vi "vipbBuild.vi"() -> ()   [LabVIEW 2014, in "lv-cli-steps.lvlib"]
uses:
  lv-cli-steps.lvlib
  <vilib>/Utility/error.llb/DialogType.ctl
  <vilib>/Wiresmith Technology/LabVIEW CLI/CLI Class/CLI.lvclass
  <vilib>/JKI/VIPM API/VIPM API_vipm_api.lvlib
panel:
  out "error out":errorcluster
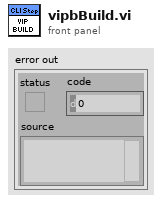
[diagram p1: front panel]
types:
  T1 = typedef "DialogType.ctl" = u16
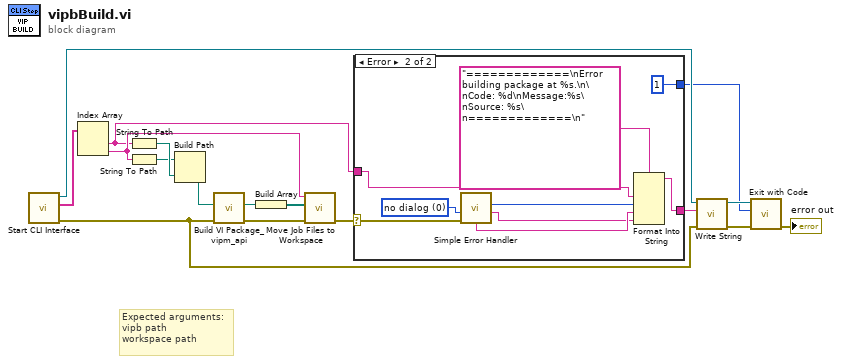
[diagram p0: block diagram]
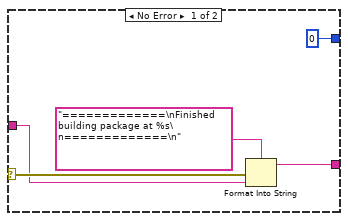
[diagram p2: hidden frame]
diagram:
  # "Expected arguments:\nvipb path\nworkspace path"
  n1 = call <vilib>:"Start CLI Interface.vi"() -> ("error out"=w3:errorcluster, "Custom Parameters"=w17:string[], "CLI out"=w15:refnum<class "CLI.lvclass">)  [unwired: 9 in]
  n2 = Index Array(array=w17) -> (element #1=w1:string, element #2=w7:string)  [unwired: 2 in]
  n3 = String To Path(string=w1) -> (path=w11:path)
  n4 = String To Path(string=w7) -> (path=w10:path)
  n5 = Build Path(base path=w10, name or relative path=w11) -> (appended path=w2:path)
  n6 = call <vilib>:"Build VI Package_vipm_api.vi"("error in (no error)"=w3, "Path to VIPB File"=w2) -> ("error out"=w4:errorcluster, "Build Output"=w6:path)  [unwired: 8 in]
  n7 = Build Array(w6) -> (w5:path[])
  n8 = call "Move Job Files to Workspace.vi"("error in (no error)"=w4, "Generated Files"=w5, "Workspace Path"=w7) -> ("error out"=w9:errorcluster)  [unwired: 8 in]
  n9 = case shown="Error" w9 {
    selector: w9 -> [w21 w30]
    tunnel: w1 -> [w20 w26]
    tunnel: [w19 w31] -> w16
    tunnel: [0 ("Exit Code (0)") 1 ("Exit Code (0)")] -> w12
    frame No Error {
      n10 = Format Into String(format string="=============\nFinished building package at %s\n=============\n", error in=w21, w20) -> (resulting string=w19:string)  [unwired: 1 in, 1 out]
    }
    frame Error {
      w29 = T1 0 items=["no dialog", "OK message", "continue or stop message", "OK message + warnings", "continue/stop + warnings"] ("type of dialog (OK msg:1)")
      n11 = call <vilib>:"Simple Error Handler.vi"("type of dialog (OK msg:1)"=w29, "error in (no error)"=w30) -> ("code out"=w23:i32, "source out"=w24:string, "message"=w25:string)  [unwired: 3 in, 2 out]
      n12 = Format Into String(format string="=============\nError building package at %s.\n\nCode: %d\nMessage:%s\nSource: %s\n=============\n", w26, w23, w25, w24) -> (resulting string=w31:string)  [unwired: 2 in, 1 out]
    }
  }
  n13 = call <vilib>:"Write String.vi"("error in (no error)"=w3, "Text to Write"=w16, "CLI in"=w15) -> ("error out"=w14:errorcluster, "CLI out"=w13:refnum<class "CLI.lvclass">)  [unwired: 7 in]
  n14 = call <vilib>:"Exit with Code.vi"("error in (no error)"=w14, "Exit Code (0)"=w12, "CLI in"=w13) -> ("error out"=→"error out":errorcluster)  [unwired: 8 in]
